vi "SIOSIfmClose.vi"   [LabVIEW 2009]
uses:
  siosifm.dll
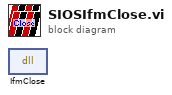
[diagram p0: block diagram]
diagram:
  n1 = dll-call lib="D:/Support/Labview/RE-10/SIOS_IfmDLL/siosifm.dll" fn="IfmClose"() -> ()  [unwired: 4 in, 2 out]
